vi "Decode (DBDE) (x8) (SubVI).vi"() -> (0 "Output Valid":bool, 3 "Data Out":u64)   [LabVIEW 2015]
uses:
  Uncompression States.ctl
  <vilib>/rvi/interface/RandomDataEmulation/niFpgaRandomDataHandleErrors.vi
  <vilib>/rvi/DataTransferAndStorage/Container/XNode/niFpgaContainer.xnode
  <vilib>/rvi/interface/RandomDataEmulation/nirviRandomDataFpgaReadWriteTemplate.vi
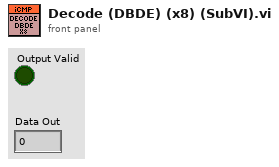
[diagram p1: front panel]
types:
  T1 = typedef "Uncompression States.ctl" = enum16{"Read BD-MIN", "Read IMG DATA", "Send Block Data"}
  T2 = cluster{"Numeric Control":u8, "Numeric Control":u8, "Numeric Control":u8, "Numeric Control":u8, "Numeric Control":u8, "Numeric Control":u8, "Numeric Control":u8, "Numeric Control":u8}
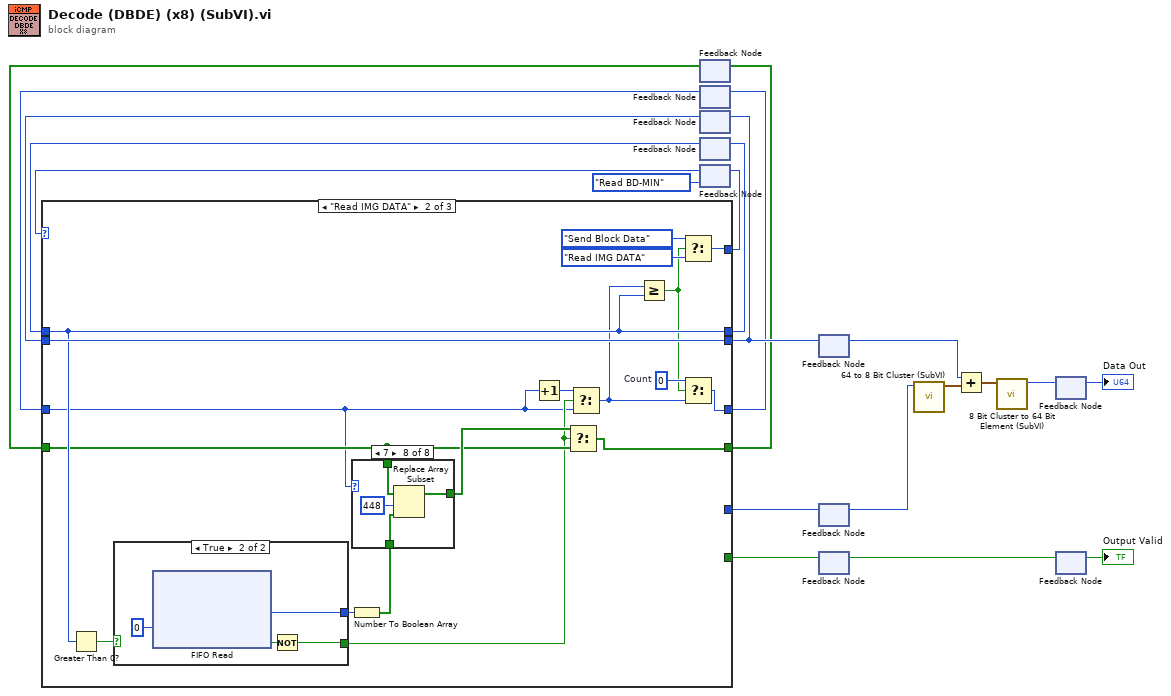
[diagram p0: block diagram]
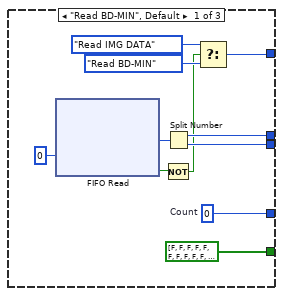
[diagram p2: hidden frame]
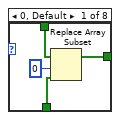
[diagram p3: hidden frame]
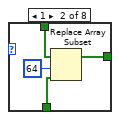
[diagram p4: hidden frame]
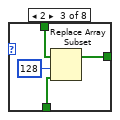
[diagram p5: hidden frame]
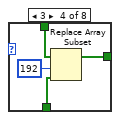
[diagram p6: hidden frame]
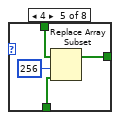
[diagram p7: hidden frame]
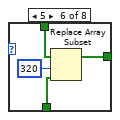
[diagram p8: hidden frame]
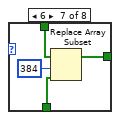
[diagram p9: hidden frame]
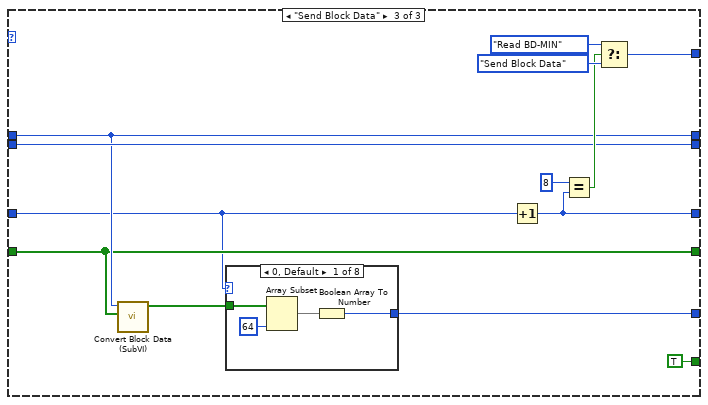
[diagram p11: hidden frame]
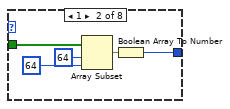
[diagram p12: hidden frame]
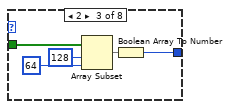
[diagram p13: hidden frame]
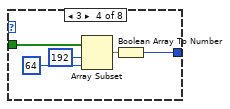
[diagram p14: hidden frame]
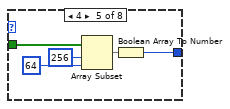
[diagram p15: hidden frame]
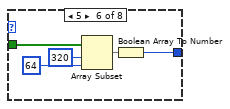
[diagram p16: hidden frame]
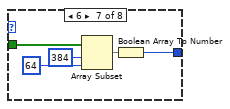
[diagram p17: hidden frame]
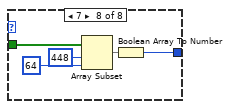
[diagram p18: hidden frame]
diagram:
  n1 = feedback #1() -> (w15:bool[])  [unwired: 1 in]
  n2 = feedback #2() -> (w17:u8)  [unwired: 1 in]
  n3 = feedback #3() -> (w14:u8)  [unwired: 1 in]
  n4 = feedback #4() -> (w13:u8)  [unwired: 1 in]
  n5 = feedback #5(Uncompression_States."Read BD-MIN") -> (w11:T1)
  n6 = case shown="\"Read IMG DATA\"" w11 {
    tunnel: [w29 w44 w95] -> w10
    tunnel: [w31 w47 w90] -> w18
    tunnel: [w30 w50 w92] -> w19
    tunnel: w13 -> [_ w47 w90]
    tunnel: w14 -> [_ w50 w92]
    tunnel: [bool[] [FALSE, FALSE, FALSE, FALSE, FALSE, FALSE, FALSE, FALSE, FALSE, FALSE, FALSE, FALSE, FALSE, FALSE, FALSE, FALSE, FALSE, FALSE, FALSE, FALSE, FALSE, FALSE, FALSE, FALSE, FALSE, FALSE, FALSE, FALSE, FALSE, FALSE, FALSE, FALSE, FALSE, FALSE, FALSE, FALSE, FALSE, FALSE, FALSE, FALSE, FALSE, FALSE, FALSE, FALSE, FALSE, FALSE, FALSE, FALSE, FALSE, FALSE, FALSE, FALSE, FALSE, FALSE, FALSE, FALSE, FALSE, FALSE, FALSE, FALSE, FALSE, FALSE, FALSE, FALSE, FALSE, FALSE, FALSE, FALSE, FALSE, FALSE, FALSE, FALSE, FALSE, FALSE, FALSE, FALSE, FALSE, FALSE, FALSE, FALSE, FALSE, FALSE, FALSE, FALSE, FALSE, FALSE, FALSE, FALSE, FALSE, FALSE, FALSE, FALSE, FALSE, FALSE, FALSE, FALSE, FALSE, FALSE, FALSE, FALSE, FALSE, FALSE, FALSE, FALSE, FALSE, FALSE, FALSE, FALSE, FALSE, FALSE, FALSE, FALSE, FALSE, FALSE, FALSE, FALSE, FALSE, FALSE, FALSE, FALSE, FALSE, FALSE, FALSE, FALSE, FALSE, FALSE, FALSE, FALSE, FALSE, FALSE, FALSE, FALSE, FALSE, FALSE, FALSE, FALSE, FALSE, FALSE, FALSE, FALSE, FALSE, FALSE, FALSE, FALSE, FALSE, FALSE, FALSE, FALSE, FALSE, FALSE, FALSE, FALSE, FALSE, FALSE, FALSE, FALSE, FALSE, FALSE, FALSE, FALSE, FALSE, FALSE, FALSE, FALSE, FALSE, FALSE, FALSE, FALSE, FALSE, FALSE, FALSE, FALSE, FALSE, FALSE, FALSE, FALSE, FALSE, FALSE, FALSE, FALSE, FALSE, FALSE, FALSE, FALSE, FALSE, FALSE, FALSE, FALSE, FALSE, FALSE, FALSE, FALSE, FALSE, FALSE, FALSE, FALSE, FALSE, FALSE, FALSE, FALSE, FALSE, FALSE, FALSE, FALSE, FALSE, FALSE, FALSE, FALSE, FALSE, FALSE, FALSE, FALSE, FALSE, FALSE, FALSE, FALSE, FALSE, FALSE, FALSE, FALSE, FALSE, FALSE, FALSE, FALSE, FALSE, FALSE, FALSE, FALSE, FALSE, FALSE, FALSE, FALSE, FALSE, FALSE, FALSE, FALSE, FALSE, FALSE, FALSE, FALSE, FALSE, FALSE, FALSE, FALSE, FALSE, FALSE, FALSE, FALSE, FALSE, FALSE, FALSE, FALSE, FALSE, FALSE, FALSE, FALSE, FALSE, FALSE, FALSE, FALSE, FALSE, FALSE, FALSE, FALSE, FALSE, FALSE, FALSE, FALSE, FALSE, FALSE, FALSE, FALSE, FALSE, FALSE, FALSE, FALSE, FALSE, FALSE, FALSE, FALSE, FALSE, FALSE, FALSE, FALSE, FALSE, FALSE, FALSE, FALSE, FALSE, FALSE, FALSE, FALSE, FALSE, FALSE, FALSE, FALSE, FALSE, FALSE, FALSE, FALSE, FALSE, FALSE, FALSE, FALSE, FALSE, FALSE, FALSE, FALSE, FALSE, FALSE, FALSE, FALSE, FALSE, FALSE, FALSE, FALSE, FALSE, FALSE, FALSE, FALSE, FALSE, FALSE, FALSE, FALSE, FALSE, FALSE, FALSE, FALSE, FALSE, FALSE, FALSE, FALSE, FALSE, FALSE, FALSE, FALSE, FALSE, FALSE, FALSE, FALSE, FALSE, FALSE, FALSE, FALSE, FALSE, FALSE, FALSE, FALSE, FALSE, FALSE, FALSE, FALSE, FALSE, FALSE, FALSE, FALSE, FALSE, FALSE, FALSE, FALSE, FALSE, FALSE, FALSE, FALSE, FALSE, FALSE, FALSE, FALSE, FALSE, FALSE, FALSE, FALSE, FALSE, FALSE, FALSE, FALSE, FALSE, FALSE, FALSE, FALSE, FALSE, FALSE, FALSE, FALSE, FALSE, FALSE, FALSE, FALSE, FALSE, FALSE, FALSE, FALSE, FALSE, FALSE, FALSE, FALSE, FALSE, FALSE, FALSE, FALSE, FALSE, FALSE, FALSE, FALSE, FALSE, FALSE, FALSE, FALSE, FALSE, FALSE, FALSE, FALSE, FALSE, FALSE, FALSE, FALSE, FALSE, FALSE, FALSE, FALSE, FALSE, FALSE, FALSE, FALSE, FALSE, FALSE, FALSE, FALSE, FALSE, FALSE, FALSE, FALSE, FALSE, FALSE, FALSE, FALSE, FALSE, FALSE, FALSE, FALSE, FALSE, FALSE, FALSE, FALSE, FALSE, FALSE, FALSE, FALSE, FALSE, FALSE, FALSE, FALSE, FALSE, FALSE, FALSE, FALSE, FALSE, FALSE, FALSE, FALSE, FALSE, FALSE, FALSE, FALSE, FALSE, FALSE, FALSE, FALSE, FALSE, FALSE, FALSE, FALSE, FALSE, FALSE, FALSE, FALSE, FALSE, FALSE, FALSE, FALSE, FALSE, FALSE, FALSE, FALSE, FALSE, FALSE, FALSE, FALSE, FALSE, FALSE, FALSE, FALSE, FALSE, FALSE, FALSE, FALSE, FALSE, FALSE, FALSE, FALSE, FALSE, FALSE, FALSE, FALSE, FALSE, FALSE, FALSE, FALSE, FALSE, FALSE, FALSE, FALSE] ("initialized array") w40 w89] -> w8
    tunnel: w15 -> [_ w38 w89]
    tunnel: [w25 w37 w99] -> w16
    tunnel: w17 -> [_ w33 w87]
    tunnel: [_ _ TRUE] -> w21
    tunnel: [_ _ w91] -> w20
    frame "Read BD-MIN", Default {
      w25 = u8 0  # Count
      n7 = xnode ("FIFO Read")("Timeout"=0) -> ("Element"=w23:u16, "Timed Out?"=w22:bool)  [unwired: 1 in, 1 out]
      n8 = Not(x=w22) -> (.not. x?=w27:bool)
      n9 = Split Number(x=w23) -> (hi(x)=w31:u8, lo(x)=w30:u8)
      n10 = Select(t=Uncompression_States."Read IMG DATA", s=w27, f=Uncompression_States."Read BD-MIN") -> (s? t:f=w29:T1)
    }
    frame "Read IMG DATA" {
      w35 = u8 0  # Count
      n11 = Greater Than 0?(x=w47) -> (x > 0?=w49:bool)
      n12 = case shown="True" w49 {
        tunnel: [_ w86] -> w36
        tunnel: [_ w83] -> w42
        frame False {
        }
        frame True {
          n13 = xnode ("FIFO Read")("Timeout"=0) -> ("Element"=w83:u64, "Timed Out?"=w84:bool)  [unwired: 1 in, 1 out]
          n14 = Not(x=w84) -> (.not. x?=w86:bool)
        }
      }
      n15 = Number To Boolean Array(number=w42) -> (Boolean array=w41:bool[])
      n16 = case shown="7" w33 {
        tunnel: w41 -> [w54 w58 w62 w66 w70 w74 w78 w82]
        tunnel: [w53 w57 w61 w65 w69 w73 w77 w81] -> w39
        tunnel: w38 -> [w52 w56 w60 w64 w68 w72 w76 w80]
        frame 0, Default {
          n17 = Replace Array Subset(array=w52, new element=w54, index=0) -> (w53:bool[])
        }
        frame 1 {
          n18 = Replace Array Subset(array=w56, new element=w58, index=64) -> (w57:bool[])
        }
        frame 2 {
          n19 = Replace Array Subset(array=w60, new element=w62, index=128) -> (w61:bool[])
        }
        frame 3 {
          n20 = Replace Array Subset(array=w64, new element=w66, index=192) -> (w65:bool[])
        }
        frame 4 {
          n21 = Replace Array Subset(array=w68, new element=w70, index=256) -> (w69:bool[])
        }
        frame 5 {
          n22 = Replace Array Subset(array=w72, new element=w74, index=320) -> (w73:bool[])
        }
        frame 6 {
          n23 = Replace Array Subset(array=w76, new element=w78, index=384) -> (w77:bool[])
        }
        frame 7 {
          n24 = Replace Array Subset(array=w80, new element=w82, index=448) -> (w81:bool[])
        }
      }
      n25 = Increment(x=w33) -> (x+1=w48:u8)
      n26 = Select(t=w39, s=w36, f=w38) -> (s? t:f=w40:bool[])
      n27 = Select(t=w48, s=w36, f=w33) -> (s? t:f=w43:u8)
      n28 = Greater Or Equal?(x=w43, y=w47) -> (x >= y?=w34:bool)
      n29 = Select(t=Uncompression_States."Send Block Data", s=w34, f=Uncompression_States."Read IMG DATA") -> (s? t:f=w44:T1)
      n30 = Select(t=w35, s=w34, f=w43) -> (s? t:f=w37:u8)
    }
    frame "Send Block Data" {
      n31 = call "Convert Block Data (SubVI).vi"("Input Array"=w89, "Bit Depth"=w90) -> ("Output Array"=w88:bool[])  [unwired: 9 in]
      n32 = case shown="0, Default" w87 {
        tunnel: [w100 w105 w110 w115 w120 w125 w130 w135] -> w91
        tunnel: w88 -> [w102 w107 w112 w117 w122 w127 w132 w137]
        frame 0, Default {
          n33 = Array Subset(array=w102, length=64) -> (w103:bool[])  [unwired: 1 in]
          n34 = Boolean Array To Number(Boolean array=w103) -> (number=w100:u64)
        }
        frame 1 {
          n35 = Array Subset(array=w107, index=64, length=64) -> (w108:bool[])
          n36 = Boolean Array To Number(Boolean array=w108) -> (number=w105:u64)
        }
        frame 2 {
          n37 = Array Subset(array=w112, index=128, length=64) -> (w113:bool[])
          n38 = Boolean Array To Number(Boolean array=w113) -> (number=w110:u64)
        }
        frame 3 {
          n39 = Array Subset(array=w117, index=192, length=64) -> (w118:bool[])
          n40 = Boolean Array To Number(Boolean array=w118) -> (number=w115:u64)
        }
        frame 4 {
          n41 = Array Subset(array=w122, index=256, length=64) -> (w123:bool[])
          n42 = Boolean Array To Number(Boolean array=w123) -> (number=w120:u64)
        }
        frame 5 {
          n43 = Array Subset(array=w127, index=320, length=64) -> (w128:bool[])
          n44 = Boolean Array To Number(Boolean array=w128) -> (number=w125:u64)
        }
        frame 6 {
          n45 = Array Subset(array=w132, index=384, length=64) -> (w133:bool[])
          n46 = Boolean Array To Number(Boolean array=w133) -> (number=w130:u64)
        }
        frame 7 {
          n47 = Array Subset(array=w137, index=448, length=64) -> (w138:bool[])
          n48 = Boolean Array To Number(Boolean array=w138) -> (number=w135:u64)
        }
      }
      n49 = Increment(x=w87) -> (x+1=w99:u8)
      n50 = Equal?(x=u8 8, y=w99) -> (x = y?=w94:bool)
      n51 = Select(t=Uncompression_States."Read BD-MIN", s=w94, f=Uncompression_States."Send Block Data") -> (s? t:f=w95:T1)
    }
  }
  n52 = feedback-in #1(w8) -> ()
  n53 = feedback-in #2(w16) -> ()
  n54 = feedback-in #3(w19) -> ()
  n55 = feedback-in #4(w18) -> ()
  n56 = feedback-in #5(w10) -> ()
  n57 = feedback-in #6(w19) -> ()
  n58 = feedback #6() -> (w5:u8)  [unwired: 1 in]
  n59 = feedback-in #7(w20) -> ()
  n60 = feedback #7() -> (w7:u64)  [unwired: 1 in]
  n61 = feedback-in #8(w21) -> ()
  n62 = feedback #8() -> (w9:bool)  [unwired: 1 in]
  n63 = call "64 to 8 Bit Cluster (SubVI).vi"("Data In"=w7) -> ("Data Out"=w6:T2)  [unwired: 10 in]
  n64 = Add(x=w5, y=w6) -> (x+y=w4:T2)
  n65 = call "8 Bit Cluster to 64 Bit Element (SubVI).vi"("Pixel Cluster"=w4) -> ("Pixel Data (64-Bit)"=w3:u64)  [unwired: 10 in]
  n66 = feedback-in #9(w3) -> ()
  n67 = feedback #9() -> (→"Data Out":u64)  [unwired: 1 in]
  n68 = feedback-in #10(w9) -> ()
  n69 = feedback #10() -> (→"Output Valid":bool)  [unwired: 1 in]
